vi "Convert Variant Parameters to TSD.vi"(9 "error in":errorcluster, 10 "Variant Parameter Array":variant[](array[variant])) -> (1 "error out":errorcluster, 2 "TestSetDef":T1)   [LabVIEW 2011]
uses:
  Test Set Definition.ctl
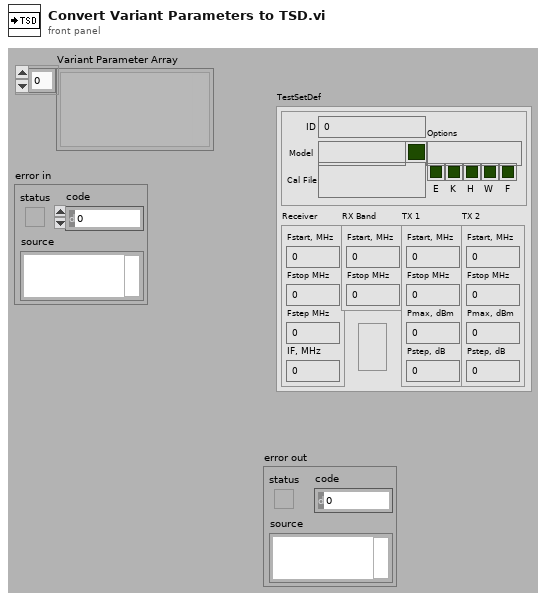
[diagram p1: front panel]
types:
  T1 = typedef "Test Set Definition.ctl" = cluster{"General":cluster{"ID":u32, "Model":string, "Dual Port?":bool, "Options":string, "Options":cluster{"E":bool, "K":bool, "H":bool, "W":bool, "F":bool}, "Cal File":path}, "Receiver":cluster{"Fstart, MHz":dbl, "Fstop MHz":dbl, "Fstep MHz":dbl, "IF, MHz":dbl}, "RX Band":cluster{"Fstart, MHz":dbl, "Fstop MHz":dbl}, "TX 1":cluster{"Fstart, MHz":dbl, "Fstop MHz":dbl, "Pmax, dBm":dbl, "Pstep, dB":dbl}, "TX 2":cluster{"Fstart, MHz":dbl, "Fstop MHz":dbl, "Pmax, dBm":dbl, "Pstep, dB":dbl}, "Low-side?":bool}
  T2 = cluster{"ID":u32, "Model":string, "Dual Port?":bool, "Options":string, "Options":cluster{"E":bool, "K":bool, "H":bool, "W":bool, "F":bool}, "Cal File":path}
  T3 = cluster{"Fstart, MHz":dbl, "Fstop MHz":dbl, "Fstep MHz":dbl, "IF, MHz":dbl}
  T4 = cluster{"Fstart, MHz":dbl, "Fstop MHz":dbl, "Pmax, dBm":dbl, "Pstep, dB":dbl}
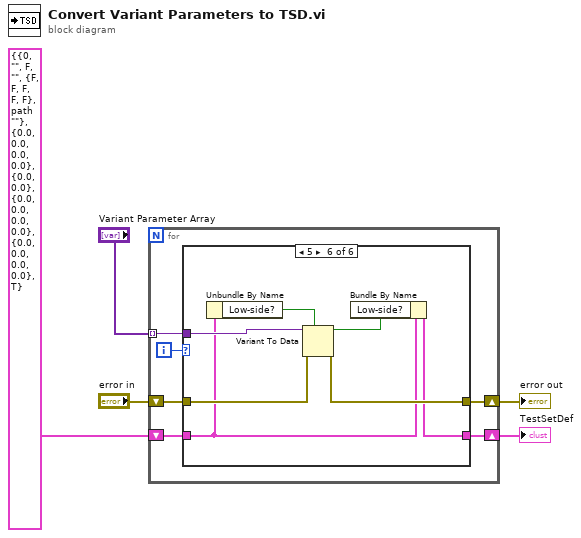
[diagram p0: block diagram]
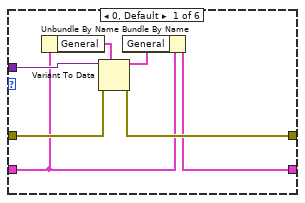
[diagram p2: hidden frame]
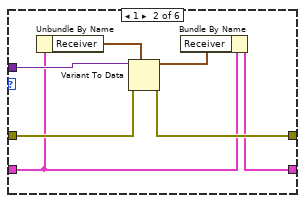
[diagram p3: hidden frame]
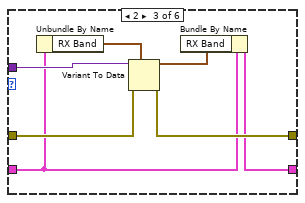
[diagram p4: hidden frame]
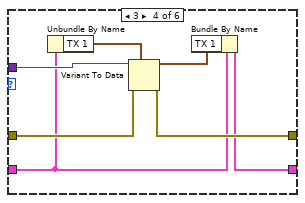
[diagram p5: hidden frame]
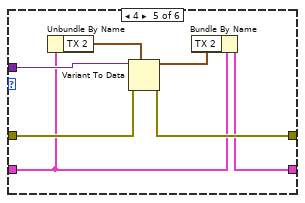
[diagram p6: hidden frame]
diagram:
  n1 = for {
    shift-right: [w10] -> w4
    shift-left: "error in" -> [w11]
    shift-right: [w7] -> w2
    shift-left: T1 {"General"={"ID"=0, "Model"="", "Dual Port?"=FALSE, "Options"="", "Options"={"E"=FALSE, "K"=FALSE, "H"=FALSE, "W"=FALSE, "F"=FALSE}, "Cal File"=path ""}, "Receiver"={"Fstart, MHz"=0.0, "Fstop MHz"=0.0, "Fstep MHz"=0.0, "IF, MHz"=0.0}, "RX Band"={"Fstart, MHz"=0.0, "Fstop MHz"=0.0}, "TX 1"={"Fstart, MHz"=0.0, "Fstop MHz"=0.0, "Pmax, dBm"=0.0, "Pstep, dB"=0.0}, "TX 2"={"Fstart, MHz"=0.0, "Fstop MHz"=0.0, "Pmax, dBm"=0.0, "Pstep, dB"=0.0}, "Low-side?"=TRUE} ("TestSetDef") -> [w8]
    tunnel: "Variant Parameter Array" -> [w9] mode=indexing
    i -> [w6]
    n2 = case shown="5" w6 {
      tunnel: w11 -> [w18 w25 w32 w39 w46 w53]
      tunnel: [w17 w24 w31 w38 w45 w52] -> w10
      tunnel: w9 -> [w16 w23 w30 w37 w44 w51]
      tunnel: w8 -> [w13 w20 w27 w34 w41 w48]
      tunnel: [w12 w19 w26 w33 w40 w47] -> w7
      frame 0, Default {
        n3 = Unbundle By Name(w13) -> ("General"=w15:T2)
        n4 = Variant To Data(error in=w18, type=w15, Variant=w16) -> (data=w14:T2, error out=w17:errorcluster)
        n5 = Bundle By Name(cluster=w13, "General"=w14) -> (w12:T1)
      }
      frame 1 {
        n6 = Unbundle By Name(w20) -> ("Receiver"=w22:T3)
        n7 = Variant To Data(error in=w25, type=w22, Variant=w23) -> (data=w21:T3, error out=w24:errorcluster)
        n8 = Bundle By Name(cluster=w20, "Receiver"=w21) -> (w19:T1)
      }
      frame 2 {
        n9 = Unbundle By Name(w27) -> ("RX Band"=w29:cluster{"Fstart, MHz":dbl, "Fstop MHz":dbl})
        n10 = Variant To Data(error in=w32, type=w29, Variant=w30) -> (data=w28:cluster{"Fstart, MHz":dbl, "Fstop MHz":dbl}, error out=w31:errorcluster)
        n11 = Bundle By Name(cluster=w27, "RX Band"=w28) -> (w26:T1)
      }
      frame 3 {
        n12 = Unbundle By Name(w34) -> ("TX 1"=w36:T4)
        n13 = Variant To Data(error in=w39, type=w36, Variant=w37) -> (data=w35:T4, error out=w38:errorcluster)
        n14 = Bundle By Name(cluster=w34, "TX 1"=w35) -> (w33:T1)
      }
      frame 4 {
        n15 = Unbundle By Name(w41) -> ("TX 2"=w43:T4)
        n16 = Variant To Data(error in=w46, type=w43, Variant=w44) -> (data=w42:T4, error out=w45:errorcluster)
        n17 = Bundle By Name(cluster=w41, "TX 2"=w42) -> (w40:T1)
      }
      frame 5 {
        n18 = Unbundle By Name(w48) -> ("Low-side?"=w50:bool)
        n19 = Variant To Data(error in=w53, type=w50, Variant=w51) -> (data=w49:bool, error out=w52:errorcluster)
        n20 = Bundle By Name(cluster=w48, "Low-side?"=w49) -> (w47:T1)
      }
    }
  }
  "error out" <- w4
  "TestSetDef" <- w2
